vi "DSF.Engine.Framework.Tx.Async.vi"(8 "error in (no error)":errorcluster, 11 "Framework in":refnum<class "DSF.Engine.Framework.lvclass">) -> (0 "error out":errorcluster, 3 "Framework out":refnum<class "DSF.Engine.Framework.lvclass">)   [LabVIEW 2017, in "DSF.Engine.lvlib" / "DSF.Engine.Framework.lvclass"]
uses:
  DSF.Engine.Framework.lvclass
  DSF.Engine.Framework.lvclass/DSF.Engine.Framework.ctl
  State/Framework State.lvclass/Framework State.ctl
  State/Framework State.lvclass
  Plugin/DSF.Engine.Plugin.lvclass
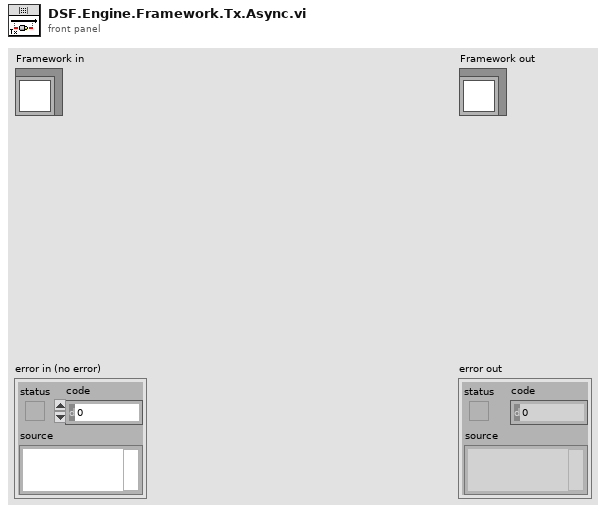
[diagram p1: front panel]
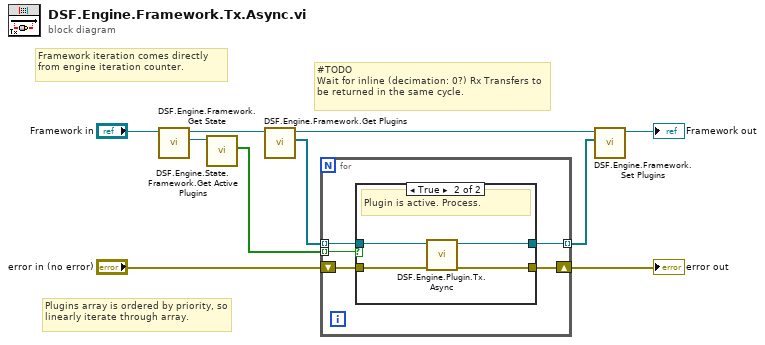
[diagram p0: block diagram]
diagram:
  # "#TODO\nWait for inline (decimation: 0?) Rx Transfers to be returned in the same cycle."
  # "Framework iteration comes directly from engine iteration counter."
  # "Plugins array is ordered by priority, so linearly iterate through array."
  n1 = call "DSF.Engine.Framework.Get State.vi"("Framework in"="Framework in") -> ("State"=w4:refnum<class "Framework State.lvclass">, "Framework out"=w1:refnum<class "DSF.Engine.Framework.lvclass">)  [unwired: 9 in]
  n2 = call "DSF.Engine.State.Framework.Get Active Plugins.vi"("Framework State in"=w4) -> ("Active Plugins"=w2:bool[])  [unwired: 9 in, 1 out]
  n3 = call "DSF.Engine.Framework.Get Plugins.vi"("Framework in"=w1) -> ("Plugins"=w10:refnum<class "DSF.Engine.Plugin.lvclass">[], "Framework out"=w5:refnum<class "DSF.Engine.Framework.lvclass">)  [unwired: 9 in]
  n4 = for {
    tunnel: w10 -> [w11] mode=indexing
    tunnel: [w15] -> w8 mode=indexing
    shift-right: [w14] -> w6
    shift-left: "error in (no error)" -> [w13]
    tunnel: w2 -> [w12] mode=indexing
    n5 = case shown="True" w12 {
      tunnel: w11 -> [w17 w21]
      tunnel: [w17 w20] -> w15
      tunnel: [w16 w18] -> w14
      tunnel: w13 -> [w16 w19]
      frame False {
        # "Plugin is not active. Skip."
      }
      frame True {
        # "Plugin is active. Process."
        n6 = call "DSF.Engine.Plugin.Tx.Async.vi"("error in (no error)"=w19, "Plugin in"=w21) -> ("error out"=w18:errorcluster, "Plugin out"=w20:refnum<class "DSF.Engine.Plugin.lvclass">)  [unwired: 8 in]
      }
    }
  }
  "error out" <- w6
  n7 = call "DSF.Engine.Framework.Set Plugins.vi"("Plugins"=w8, "Framework in"=w5) -> ("Framework out"=→"Framework out":refnum<class "DSF.Engine.Framework.lvclass">)  [unwired: 9 in]
